vi "NoLaterate.vi"(0 "Old Coords":T1 {"Angle" format="%#_13g"}) -> (1 "x out":dbl, 2 "y out":dbl)   [LabVIEW 2015]
uses:
  <vilib>/Analysis/coordinate.llb/2D Cartesian Coordinate Shift (Scalar).vi
  <vilib>/Analysis/NI_AALPro.lvlib
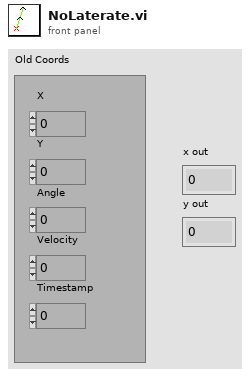
[diagram p1: front panel]
types:
  T1 = cluster{"X":dbl, "Y":dbl, "Angle":dbl, "Velocity":dbl, "Timestamp":u32}
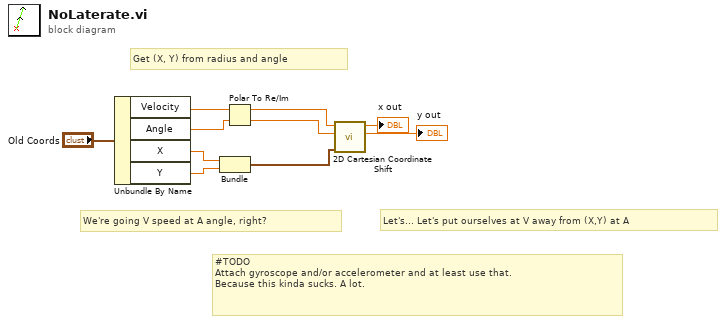
[diagram p0: block diagram]
diagram:
  # "#TODO\nAttach gyroscope and/or accelerometer and at least use that.\nBecause this kinda sucks. A lot."
  # "Get (X, Y) from radius and angle"
  # "Let's... Let's put ourselves at V away from (X,Y) at A"
  # "We're going V speed at A angle, right?"
  n1 = Unbundle By Name("Old Coords") -> ("Velocity"=w7:dbl, "Angle"=w6:dbl, "X"=w9:dbl, "Y"=w8:dbl)
  n2 = Bundle("X"=w9, "Y"=w8) -> (w5:cluster{"X":dbl, "Y":dbl})  [unwired: 1 in]
  n3 = Polar To Re/Im(2:w6, 3:w7) -> (0:w3:dbl, 1:w4:dbl)
  n4 = call-poly <vilib>:"2D Cartesian Coordinate Shift.vi"("shift"=w5, "y"=w3, "x"=w4) -> ("y out"=→"y out":dbl, "x out"=→"x out":dbl)  [unwired: 6 in, 1 out]
